vi "Enqueue.vi"(5 "subchannel":i32, 6 "abort? (F)":bool, 7 "last element? (F)":bool, 8 "element":cluster{"cmd":string, "data":variant}, 9 "event priority":T1=enum."normal priority", 10 "is valid? (T)":bool=TRUE, 11 "data in":refnum<class "EventMessengerMData.lvclass">) -> (0 "last element?":bool, 3 "data out":refnum<class "EventMessengerMData.lvclass">, 4 "aborted?":bool)   [LabVIEW 2019, in "Event MessengerM.lvlib" / "EventMessengerMData.lvclass"]
uses:
  EventMessengerMData.lvclass
  EventMessengerMData.lvclass/EventMessengerMData.ctl
  <vilib>/event_ctls.llb/usereventprio.ctl
  Event Data.ctl
  Event MessengerM.lvlib
  <vilib>/Utility/miscctls.llb/LVMapReplaceAction.ctl
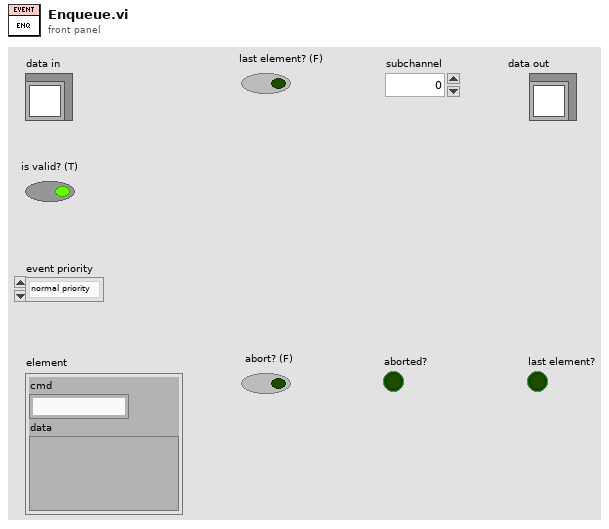
[diagram p1: front panel]
types:
  T1 = typedef "usereventprio.ctl" = enum32{"high priority", "normal priority"}
  T2 = typedef "LVMapReplaceAction.ctl" = enum32{"Modify Entry only if found", "Add or Modify Entry", "Delete Entry"}
  T3 = map{i32, cluster{"Write Count":u32, "Reg Refnum":u32, "aborted?":bool, "last element?":bool, "Event Refnum":refnum<user-event>}}
  T4 = cluster{"Write Count":u32, "Reg Refnum":u32, "aborted?":bool, "last element?":bool, "Event Refnum":refnum<user-event>}
  T5 = typedef "Event MessengerM.lvlib/Event Data.ctl" = cluster{"msg":cluster{"cmd":string, "data":variant}, "valid?":bool, "last?":bool, "aborted?":bool}
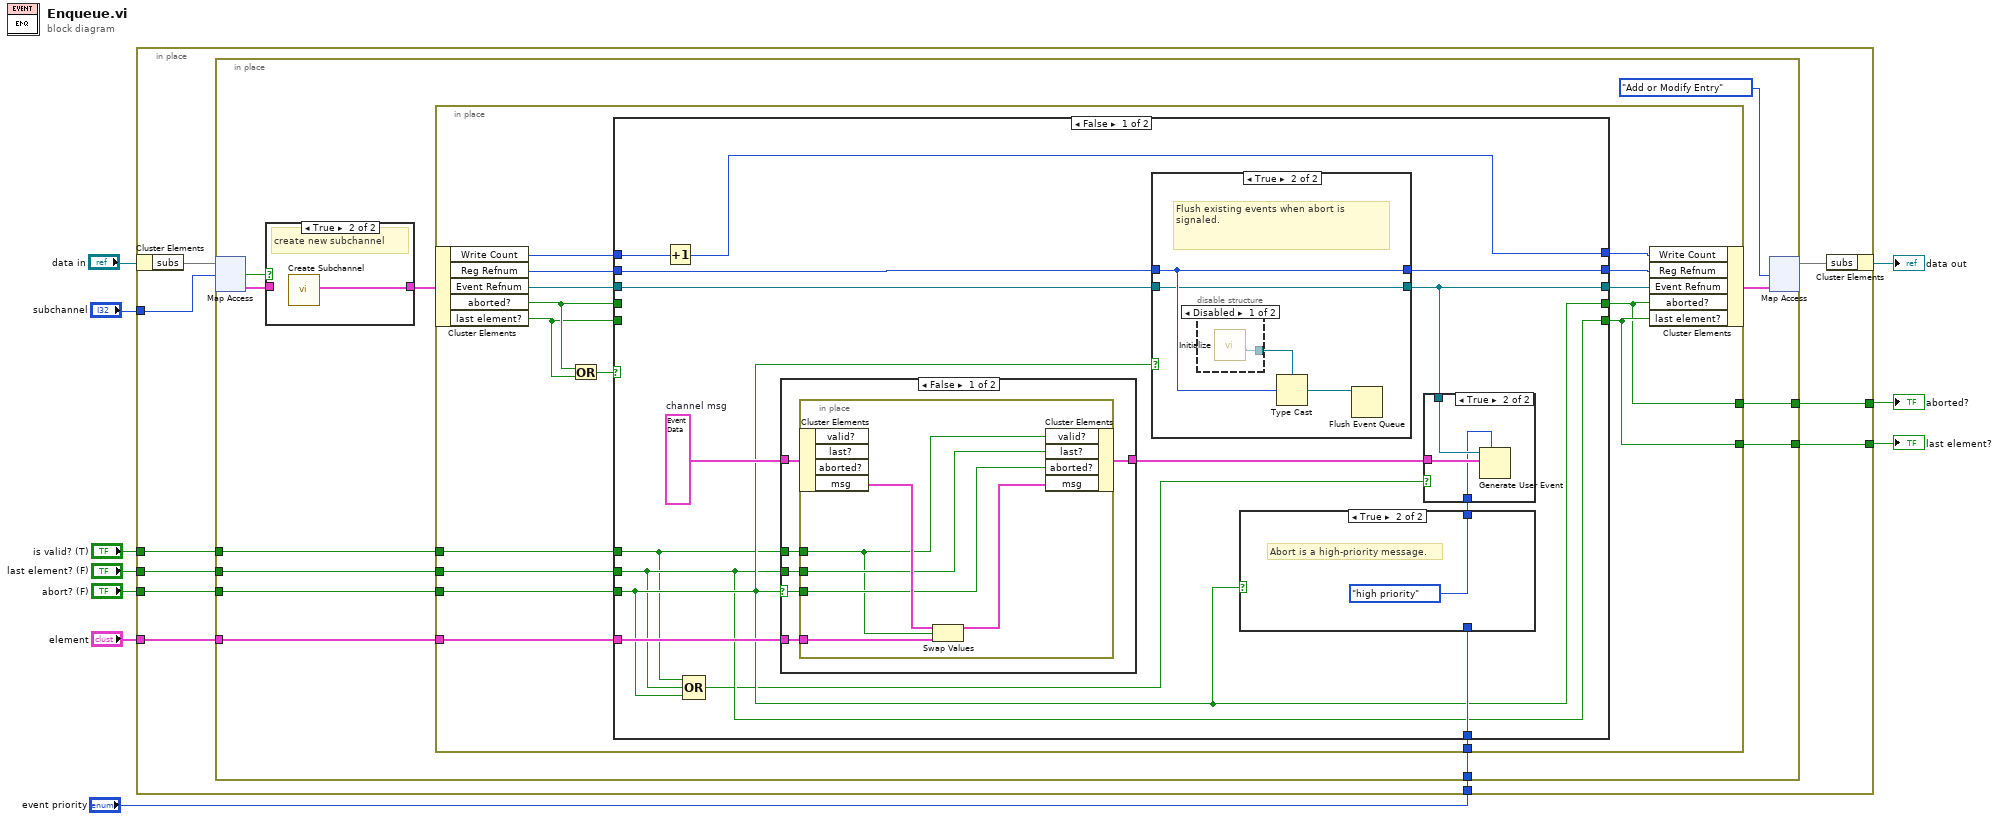
[diagram p0: block diagram]
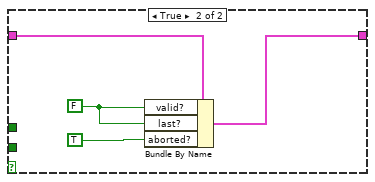
[diagram p5: hidden frame]
diagram:
  n1 = in-place {
    in-place-border: "element" -> [w20]
    in-place-border: "is valid? (T)" -> [w19]
    in-place-border: "last element? (F)" -> [w18]
    in-place-border: "abort? (F)" -> [w17]
    in-place-border: [w16] -> w6
    in-place-border: [w15] -> w5
    in-place-border: "event priority" -> [w14]
    in-place-border: "subchannel" -> [w11]
    n2 = in-place-cluster #1("data in") -> ("subs"=w13:T3)
    n3 = in-place {
      in-place-border: w20 -> [w32]
      in-place-border: w19 -> [w31]
      in-place-border: w18 -> [w30]
      in-place-border: w17 -> [w29]
      in-place-border: [w28] -> w16
      in-place-border: [w27] -> w15
      in-place-border: w14 -> [w26]
      n4 = in-place-map #2(w13, w11) -> (w24:T4, w23:bool)  [unwired: 1 in]
      n5 = case shown="True" w23 {
        tunnel: w24 -> [w33 _]
        tunnel: [w33 w34] -> w21
        frame False {
          # "subchannel exists"
        }
        frame True {
          # "create new subchannel"
          n6 = call "Create Subchannel.vi"() -> ("subchannel"=w34:T4)  [unwired: 10 in, 1 out]
        }
      }
      n7 = in-place {
        in-place-border: w32 -> [w48]
        in-place-border: w31 -> [w43]
        in-place-border: w30 -> [w42]
        in-place-border: w29 -> [w41]
        in-place-border: [w37] -> w28
        in-place-border: [w36] -> w27
        in-place-border: w26 -> [w35]
        n8 = in-place-cluster #3(w21) -> ("Write Count"=w50:u32, "Reg Refnum"=w44:u32, "Event Refnum"=w47:refnum<user-event>, "aborted?"=w39:bool, "last element?"=w38:bool)
        n9 = Or(x=w39, y=w38) -> (x .or. y?=w40:bool)
        n10 = case shown="False" w40 {
          tunnel: w50 -> [w65 w98]
          tunnel: [w64 w98] -> w49
          tunnel: w48 -> [w62 _]
          tunnel: w47 -> [w59 w96]
          tunnel: [w60 w96] -> w46
          tunnel: [w58 w97] -> w45
          tunnel: w44 -> [w63 w97]
          tunnel: [w54 w95] -> w36
          tunnel: w43 -> [w52 _]
          tunnel: w42 -> [w53 _]
          tunnel: w41 -> [w54 _]
          tunnel: w39 -> [_ w95]
          tunnel: [w53 w94] -> w37
          tunnel: w38 -> [_ w94]
          tunnel: w35 -> [w56 _]
          frame False {
            w57 = T5 {"msg"={"cmd"="", "data"=variant}, "valid?"=FALSE, "last?"=FALSE, "aborted?"=FALSE}  # channel msg
            n11 = Increment(x=w65) -> (x+1=w64:u32)
            n12 = Compound Arithmetic op=OR(w52, w53, w54) -> (w51:bool)
            n13 = case shown="False" w54 {
              selector: w54 -> [w72 _]
              tunnel: w52 -> [w76 _]
              tunnel: w62 -> [w75 _]
              tunnel: [w74 w85] -> w61
              tunnel: w57 -> [w73 w86]
              tunnel: w53 -> [w71 _]
              frame False {
                n14 = in-place {
                  in-place-border: w76 -> [w77]
                  in-place-border: w71 -> [w78]
                  in-place-border: w72 -> [w79]
                  in-place-border: w75 -> [w81]
                  n15 = in-place-cluster #4(w73) -> ("msg"=w82:cluster{"cmd":string, "data":variant})  [unwired: 3 out]
                  n16 = Swap Values(12:w82, 13:w77, 14:w81) -> (1:w80:cluster{"cmd":string, "data":variant})  [unwired: 1 out]
                  n17 = in-place-cluster #4("valid?"=w77, "last?"=w78, "aborted?"=w79, "msg"=w80) -> (w74:T5)
                }
              }
              frame True {
                w83 = FALSE ("element valid?")
                n18 = Bundle By Name(cluster=w86, "valid?"=w83, "last?"=w83, "aborted?"=TRUE ("last element?")) -> (w85:T5)
              }
            }
            n19 = case shown="True" w54 {
              tunnel: [w88 w90] -> w60
              tunnel: w59 -> [w88 w90]
              tunnel: [w87 w92] -> w58
              tunnel: w63 -> [w87 w92]
              frame False {
                # "If not aborting, keep using the same refnum as previous Write calls."
              }
              frame True {
                # "Flush existing events when abort is signaled."
                n20 = disable-structure shown="Disabled" {
                  disable-tunnel: [w93 _] -> w89
                  frame Disabled {
                    n21 = call "Initialize.vi"() -> ("Event Registration Refnum"=w93:refnum<event-registration>)  [unwired: 10 in, 1 out]
                  }
                  frame Enabled {
                  }
                }
                n22 = Type Cast(type=w89, x=w92) -> (*(type *) &x=w91:refnum<event-registration>)
                n23 = Flush Event Queue(0:w91) -> ()  [unwired: 5 in, 3 out]
              }
            }
            n24 = case shown="True" w54 {
              tunnel: w56 -> [w69 _]
              tunnel: [w69 usereventprio."high priority" ("event priority")] -> w55
              frame False {
              }
              frame True {
                # "Abort is a high-priority message."
              }
            }
            n25 = case shown="True" w51 {
              tunnel: w61 -> [_ w68]
              tunnel: w60 -> [_ w67]
              tunnel: w55 -> [_ w66]
              frame False {
              }
              frame True {
                n26 = Generate User Event(priority (normal)=w66, user event=w67, event data cluster=w68) -> ()  [unwired: 1 in, 2 out]
              }
            }
          }
          frame True {
            # "If aborted or last element has already been sent on previous writes then this channel is done until it gets re-initialized, so don't do anything now."
          }
        }
        n27 = in-place-cluster #3("Write Count"=w49, "Reg Refnum"=w45, "Event Refnum"=w46, "aborted?"=w36, "last element?"=w37) -> (w25:T4)
      }
      n28 = in-place-map #2(w25, LVMapReplaceAction."Add or Modify Entry" ("action")) -> (w12:T3)  [unwired: 2 out]
    }
    n29 = in-place-cluster #1("subs"=w12) -> (→"data out":refnum<class "EventMessengerMData.lvclass">)
  }
  "aborted?" <- w5
  "last element?" <- w6
